vi "Create Virtual Folder Hierarchy.vi"(7 "Create Sub-Bus Folder (F)":bool, 8 "error in":errorcluster, 9 "Bus Number":i32, 10 "Virtual Folder Name":string, 11 "Path to Project":path) -> (0 "error out":errorcluster, 1 "FPGA Target Found":bool, 2 "New Virtual Folder":refnum<vi>, 3 "Project:Open":refnum<vi>)   [LabVIEW 2014, in "SPI Engine Scripting.lvlib"]
doc: "Creates a specified virtual folder at the following path in the project directory: FPGA Target>>SPI Engine>> Current Bus. If the FPGA Target isn't found, an error is thrown. If either of the folders aren't found, they're created."
uses:
  SPI Engine Scripting.lvlib
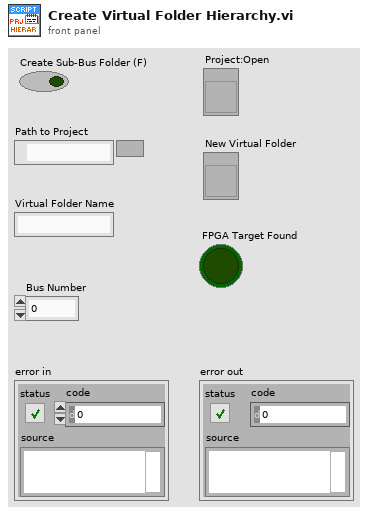
[diagram p1: front panel]
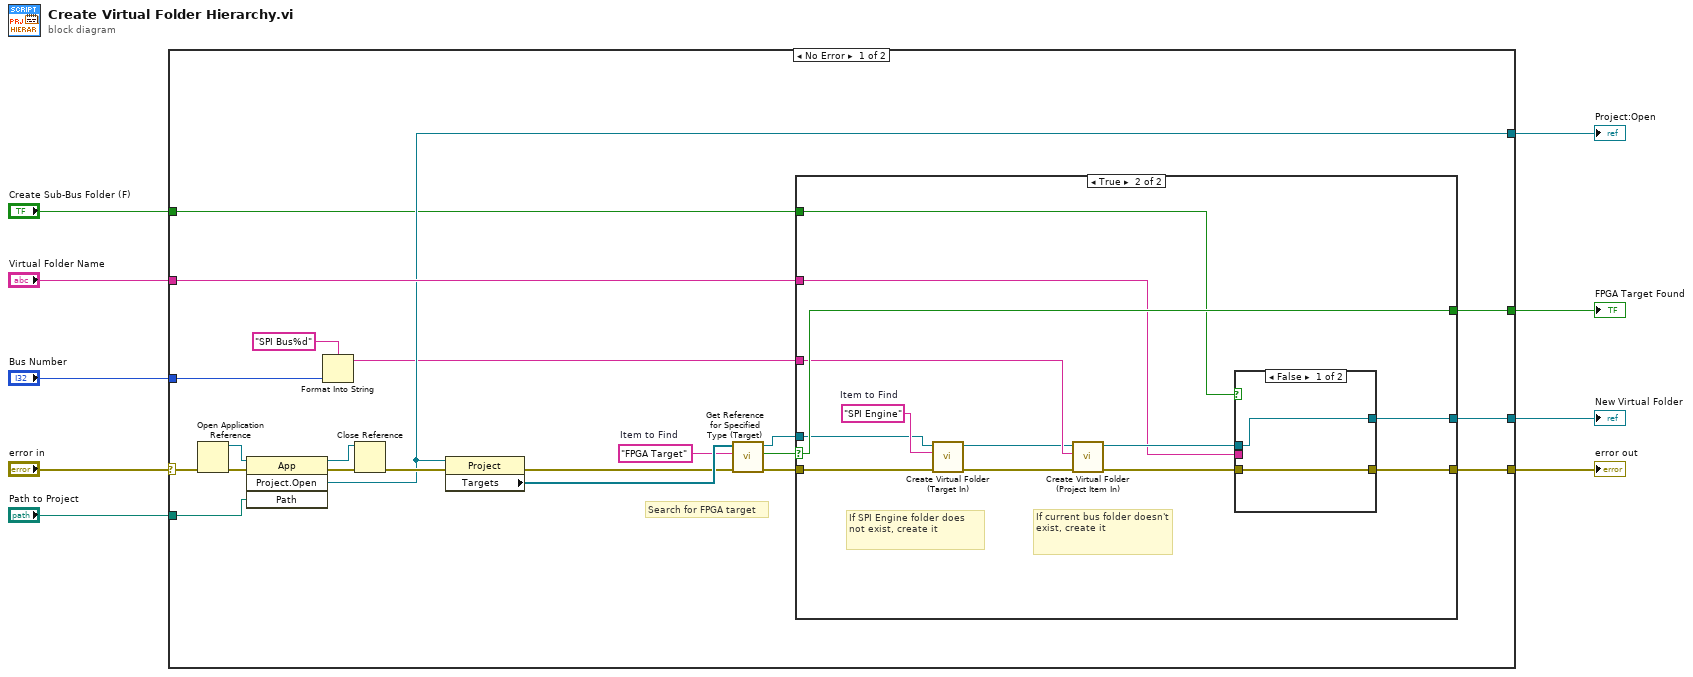
[diagram p0: block diagram]
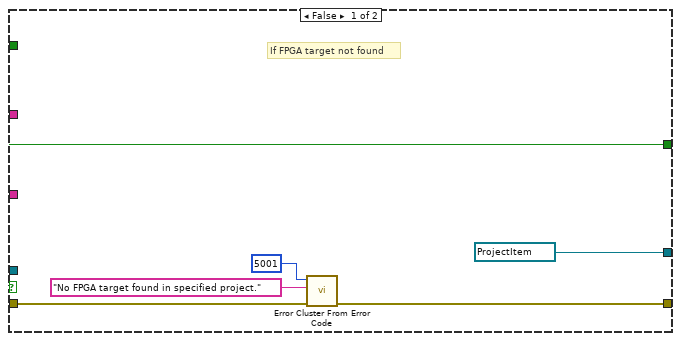
[diagram p2: hidden frame]
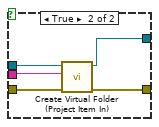
[diagram p3: hidden frame]
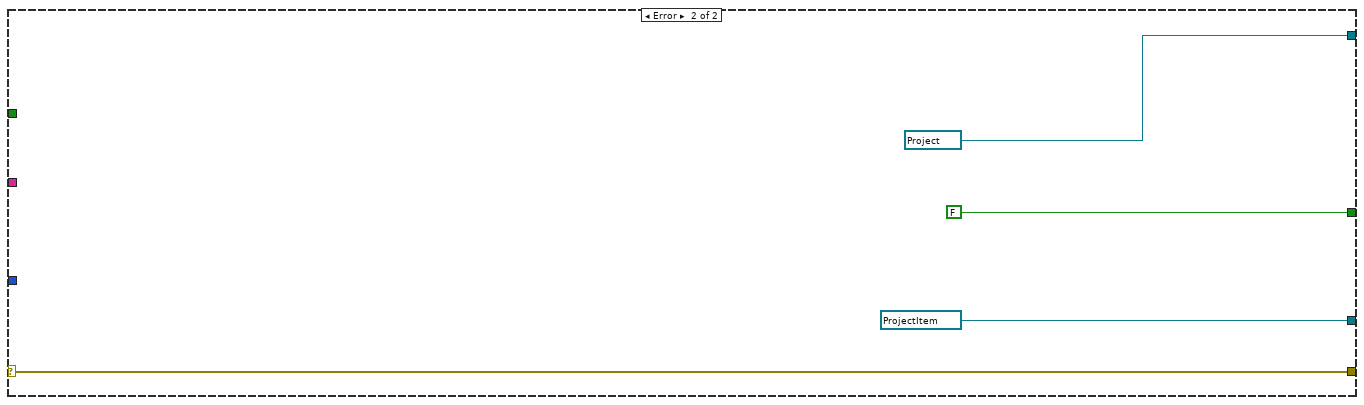
[diagram p4: hidden frame]
diagram:
  n1 = case shown="No Error" "error in" {
    selector: "error in" -> [w26 w58]
    tunnel: "Path to Project" -> [w29 _]
    tunnel: [w23 w58] -> w7
    tunnel: [w21 FALSE] -> w6
    tunnel: "Virtual Folder Name" -> [w20 _]
    tunnel: [w18 refnum<vi> refnum ("Project:Open")] -> w4
    tunnel: [w17 refnum<vi> refnum ("Project Item")] -> w3
    tunnel: "Bus Number" -> [w13 _]
    tunnel: "Create Sub-Bus Folder (F)" -> [w11 _]
    frame No Error {
      w30 = "FPGA Target"  # Item to Find
      # "Search for FPGA target"
      n2 = Open Application Reference(8:w26) -> (0:w27:errorcluster, 3:w28:refnum<vi>)  [unwired: 3 in]
      n3 = invoke class="App" method="Project.Open"(reference=w28, error in=w27, "Path"=w29) -> (reference out=w15:refnum<vi>, error out=w16:errorcluster, "Project:Open"=w18:refnum<vi>)  [unwired: 1 in, 1 out]
      n4 = Format Into String(format string="SPI Bus%d", w13) -> (resulting string=w12:string)  [unwired: 2 in, 1 out]
      n5 = Close Reference(reference=w15, error in (no error)=w16) -> (error out=w19:errorcluster)
      n6 = property class="Project"(reference=w18, error in=w19) -> (error out=w10:errorcluster, "Targets"=w31:refnum<vi>[])  [unwired: 1 out]
      n7 = call "Get Reference for Specified Type (Target).vi"("error in (no error)"=w10, "Item to Find"=w30, "Array of References"=w31) -> ("error out"=w25:errorcluster, "Item Found"=w22:bool, "TargetItem out"=w24:refnum<vi>)  [unwired: 6 in]
      n8 = case shown="True" w22 {
        selector: w22 -> [w36 w50]
        tunnel: [refnum<vi> refnum ("AddItem") w44] -> w17
        tunnel: w25 -> [w32 w41]
        tunnel: w24 -> [_ w42]
        tunnel: [w33 w45] -> w23
        tunnel: [w36 w50] -> w21
        tunnel: w20 -> [_ w46]
        tunnel: w12 -> [_ w49]
        tunnel: w11 -> [_ w38]
        frame False {
          # "If FPGA target not found"
          n9 = call <vilib>:"Error Cluster From Error Code.vi"("error in (no error)"=w32, "error message (\"\")"="No FPGA target found in specified project." ("error message (\"\")"), "error code (0)"=5001) -> ("error out"=w33:errorcluster)  [unwired: 6 in]
        }
        frame True {
          w43 = "SPI Engine"  # Item to Find
          # "If current bus folder doesn't exist, create it"
          # "If SPI Engine folder does not exist, create it"
          n10 = call "Create Virtual Folder (Target In).vi"("error in"=w41, "Item to Find"=w43, "TargetItem in"=w42) -> ("error out"=w40:errorcluster, "ProjectItem out"=w39:refnum<vi>)  [unwired: 7 in]
          n11 = call "Create Virtual Folder (Project Item In).vi"("error in"=w40, "Item to Find"=w49, "ProjectItem In"=w39) -> ("error out"=w48:errorcluster, "ProjectItem out"=w47:refnum<vi>)  [unwired: 7 in]
          n12 = case shown="False" w38 {
            tunnel: w48 -> [w51 w57]
            tunnel: w47 -> [w52 w56]
            tunnel: w46 -> [_ w55]
            tunnel: [w51 w54] -> w45
            tunnel: [w52 w53] -> w44
            frame False {
            }
            frame True {
              n13 = call "Create Virtual Folder (Project Item In).vi"("error in"=w57, "Item to Find"=w55, "ProjectItem In"=w56) -> ("error out"=w54:errorcluster, "ProjectItem out"=w53:refnum<vi>)  [unwired: 7 in]
            }
          }
        }
      }
    }
    frame Error {
    }
  }
  "error out" <- w7
  "New Virtual Folder" <- w3
  "FPGA Target Found" <- w6
  "Project:Open" <- w4
